vi "Link Parameters.vi"(7 "Virtual Memory Unit in":refnum<class "Virtual Memory Unit.lvclass">, 8 "error in (no error)":errorcluster, 11 "Remote Terminal in":refnum<class "Remote Terminal.lvclass">) -> (0 "error out":errorcluster, 3 "Remote Terminal out":refnum<class "Remote Terminal.lvclass">)   [LabVIEW 2020, in "BCI-1553 API.lvlib" / "Remote Terminal.lvclass"]
doc: "Should be the final configuration step. Actively links each parameter name to a base address that defines where the parameter may be located on the Holt IC. This is then stored in the appropriate Read/Write registries."
uses:
  Remote Terminal.lvclass
  Dependencies/Virtual Memory Unit/Virtual Memory Unit.lvclass
  Dependencies/Registry/Registry.lvclass/Registry.ctl
  Remote Terminal.lvclass/Remote Terminal.ctl
  <vilib>/Utility/error.llb/Clear Errors.vi
  Dependencies/Registry/Registry.lvclass
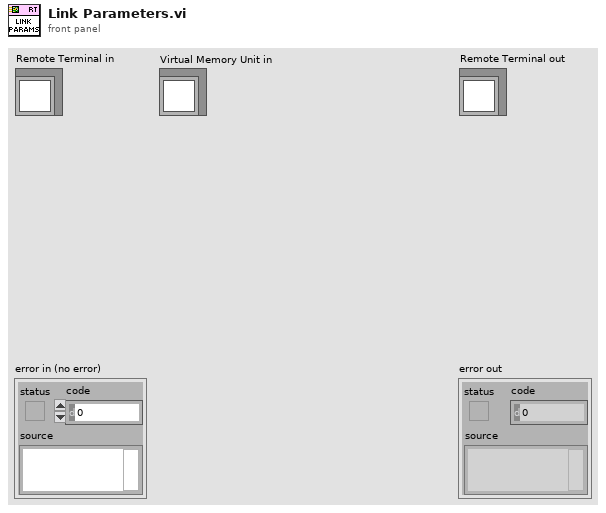
[diagram p1: front panel]
types:
  T1 = typedef "BCI-1553 API.lvlib/Remote Terminal.lvclass/RT CMD Config - Private.ctl" = cluster{"Command Type":T2, "SubAddress":T3, "Word Count\\Mode Code":T4, "Initial Data":u16[], "Data Fields":T5[]}
  T2 = typedef "BCI-1553 API.lvlib/Command Type.ctl" = enum16{"Transmit", "Receive"}
  T3 = typedef "BCI-1553 API.lvlib/Command SubAddress.ctl" = enum16{"Mode Code", "1", "2", "3", "4", "5", "6", "7", "8", "9", "10", "11", "12", "13", "14", "15", "16", "17", "18", "19", "20", "21", "22", "23", "24", "25", "26", "27", "28", "29", "30"}
  T4 = typedef "BCI-1553 API.lvlib/Command Word Count.ctl" = enum16{"1", "2", "3", "4", "5", "6", "7", "8", "9", "10", "11", "12", "13", "14", "15", "16", "17", "18", "19", "20", "21", "22", "23", "24", "25", "26", "27", "28", "29", "30", "31", "32"}
  T5 = typedef "BCI-1553 API.lvlib/Parameter Table Data.ctl" = cluster{"Parameter Name":string, "Base Word":u16, "Address":u16, "Value":u64, "Mask":u16[], "Scaling Info":T6}
  T6 = typedef "BCI-1553 API.lvlib/Scaling Information.ctl" = cluster{"Bit Offset":i32, "Bit Count":i32, "LSB Resolution":dbl, "2's Complement":bool, "Big Endian":bool, "Sign Bit":bool}
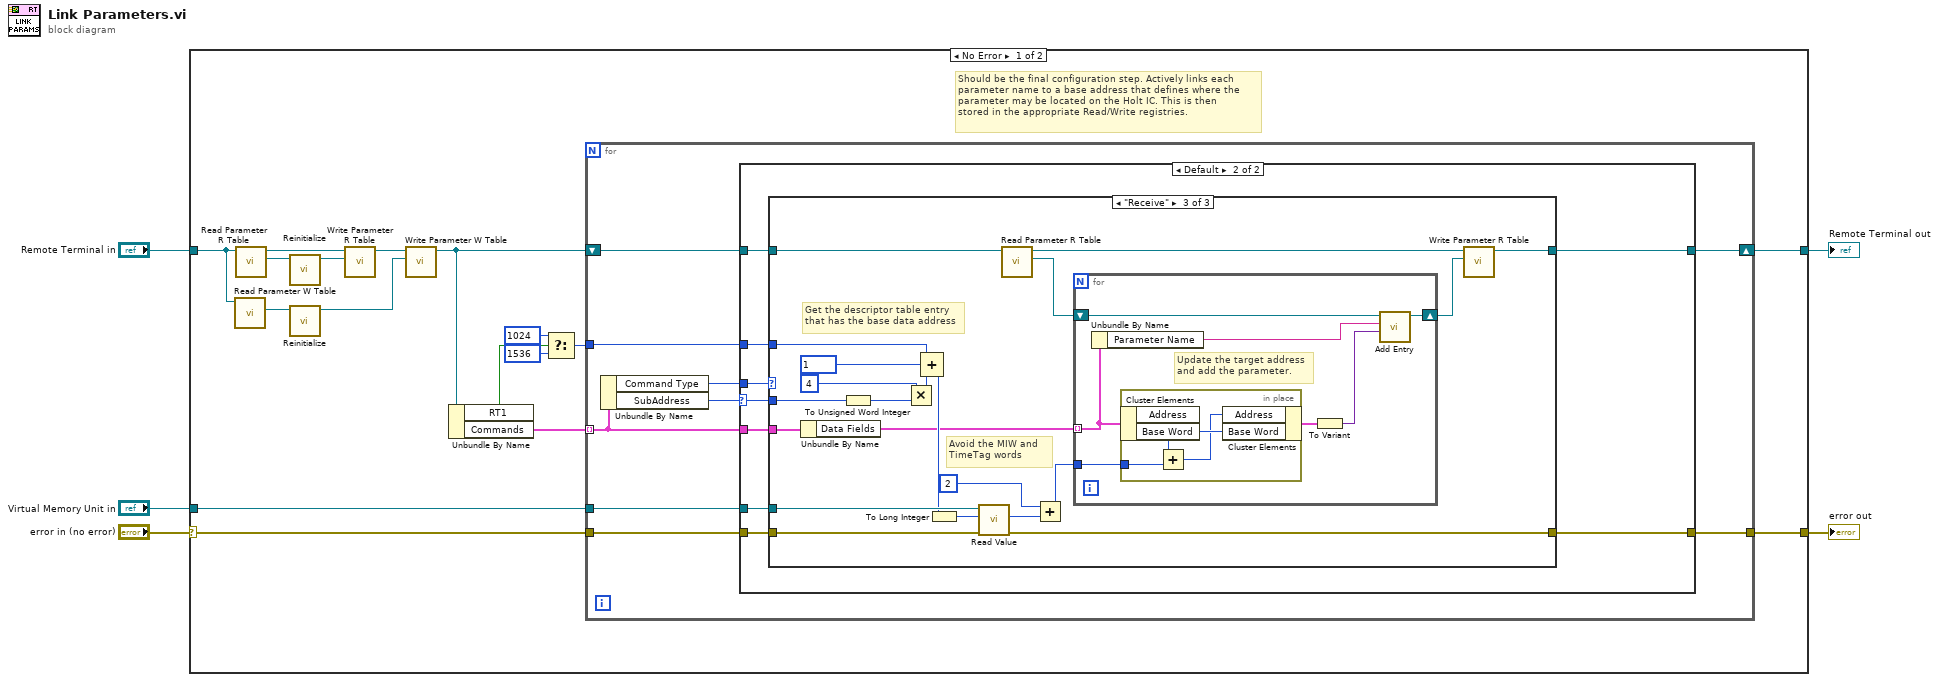
[diagram p0: block diagram]
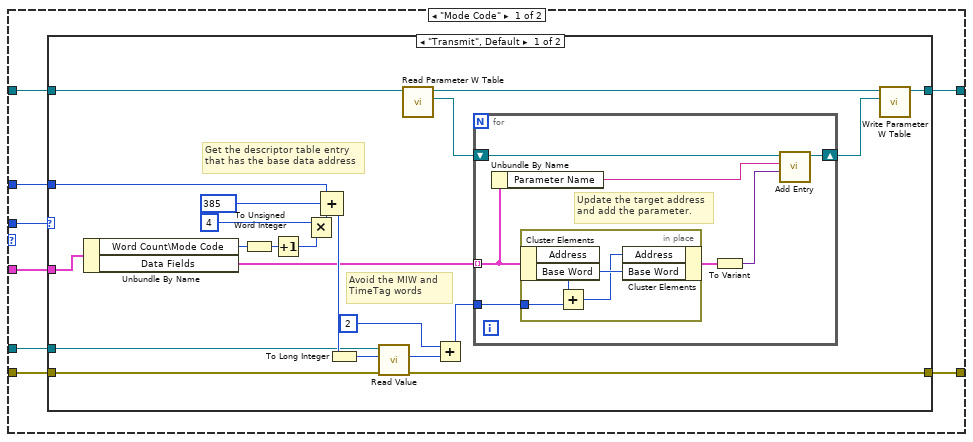
[diagram p2: hidden frame]
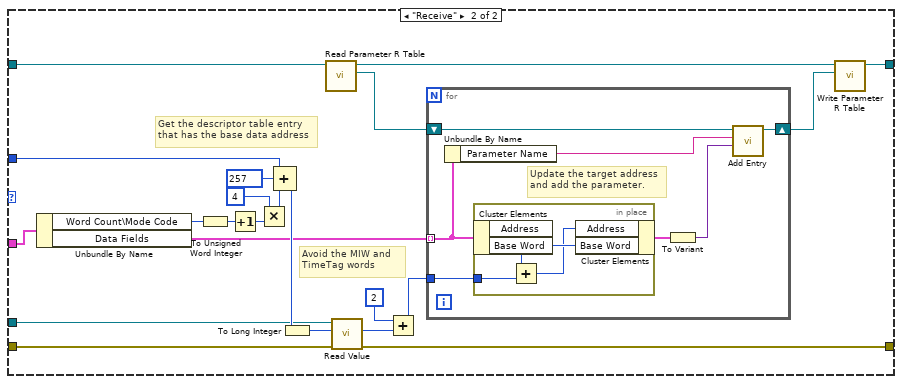
[diagram p3: hidden frame]
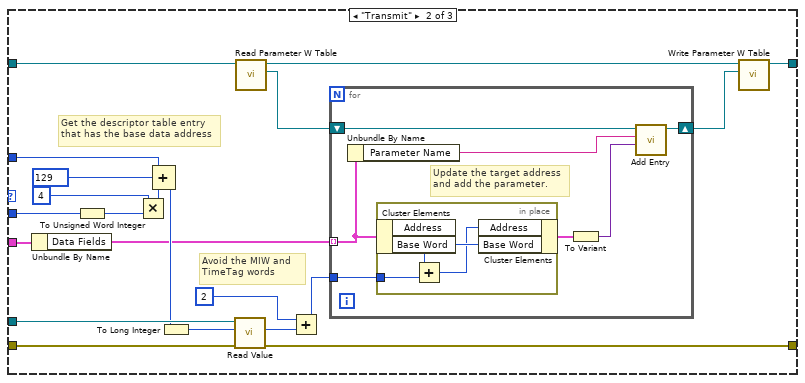
[diagram p5: hidden frame]
diagram:
  n1 = case shown="No Error" "error in (no error)" {
    selector: "error in (no error)" -> [w21 w178]
    tunnel: [w22 w178] -> w4
    tunnel: [w14 w177] -> w2
    tunnel: "Remote Terminal in" -> [w9 w177]
    tunnel: "Virtual Memory Unit in" -> [w20 _]
    frame No Error {
      # "Should be the final configuration step. Actively links each\nparameter name to a base address that defines where the\nparameter may be located on the Holt IC. This is then\nstored in the appropriate Read/Write registries."
      n2 = call-dynamic "Read Parameter W Table.vi"("1553 SubComponent in"=w9) -> ("Parameter W Table"=w10:refnum<class "Registry.lvclass">)  [unwired: 8 in, 2 out]
      n3 = call-dynamic "Read Parameter R Table.vi"("1553 SubComponent in"=w9) -> ("Parameter R Table"=w12:refnum<class "Registry.lvclass">, "1553 SubComponent out"=w13:refnum<class "Remote Terminal.lvclass">)  [unwired: 8 in, 1 out]
      n4 = call "Reinitialize.vi"("Registry in"=w12) -> ("Registry out"=w11:refnum<class "Registry.lvclass">)  [unwired: 9 in, 1 out]
      n5 = call "Reinitialize.vi"("Registry in"=w10) -> ("Registry out"=w6:refnum<class "Registry.lvclass">)  [unwired: 9 in, 1 out]
      n6 = call-dynamic "Write Parameter R Table.vi"("Parameter R Table"=w11, "1553 SubComponent in"=w13) -> ("1553 SubComponent out"=w8:refnum<class "Remote Terminal.lvclass">)  [unwired: 8 in, 1 out]
      n7 = call-dynamic "Write Parameter W Table.vi"("Parameter W Table"=w6, "1553 SubComponent in"=w8) -> ("1553 SubComponent out"=w7:refnum<class "Remote Terminal.lvclass">)  [unwired: 8 in, 1 out]
      n8 = Unbundle By Name(w7) -> ("RT1"=w15:bool, "Commands"=w19:T1[])
      n9 = Select(t=u16 1024 ("Address"), s=w15, f=u16 1536 ("Address")) -> (s? t:f=w16:u16)
      n10 = for {
        tunnel: w21 -> [w28]
        tunnel: [w29] -> w22
        tunnel: w19 -> [w30] mode=indexing
        tunnel: w16 -> [w26]
        tunnel: w20 -> [w27]
        shift-right: [w25] -> w14
        shift-left: w7 -> [w24]
        n11 = Unbundle By Name(w30) -> ("Command Type"=w31:T2, "SubAddress"=w23:T3)
        n12 = case shown="Default" w23 {
          selector: w23 -> [_ w104]
          tunnel: w31 -> [w35 w112]
          tunnel: w30 -> [w32 w111]
          tunnel: [w39 w110] -> w29
          tunnel: w28 -> [w38 w109]
          tunnel: w27 -> [w33 w108]
          tunnel: w26 -> [w34 w107]
          tunnel: [w37 w106] -> w25
          tunnel: w24 -> [w36 w105]
          frame "Mode Code" {
            n13 = case shown="\"Transmit\", Default" w35 {
              tunnel: [w42 w72] -> w39
              tunnel: w38 -> [w43 w73]
              tunnel: [w45 w75] -> w37
              tunnel: w36 -> [w46 w76]
              tunnel: w34 -> [w41 w77]
              tunnel: w33 -> [w44 w74]
              tunnel: w32 -> [w40 w78]
              frame "Transmit", Default {
                # "Get the descriptor table entry\nthat has the base data address"
                # "Avoid the MIW and\nTimeTag words"
                n14 = Unbundle By Name(w40) -> ("Word Count\\Mode Code"=w58:T4, "Data Fields"=w52:T5[])
                n15 = To Unsigned Word Integer(number=w58) -> (unsigned 16bit integer=w48:u16)
                n16 = Increment(x=w48) -> (x+1=w47:u16)
                n17 = Multiply(x=u16 4 ("y"), y=w47) -> (x*y=w59:u16)
                n18 = Compound Arithmetic op=ADD(w41, u16 385 ("Address"), w59) -> (w57:u16)
                n19 = To Long Integer(number=w57) -> (32bit integer=w56:i32)
                n20 = call "Read Value.vi"("error in (no error)"=w43, "Index"=w56, "Virtual Memory Unit in"=w44) -> ("error out"=w42:errorcluster, "Value"=w55:u16)  [unwired: 7 in]
                n21 = call-dynamic "Read Parameter W Table.vi"("1553 SubComponent in"=w46) -> ("Parameter W Table"=w50:refnum<class "Registry.lvclass">, "1553 SubComponent out"=w49:refnum<class "Remote Terminal.lvclass">)  [unwired: 8 in, 1 out]
                n22 = Add(x=u16 2 ("y"), y=w55) -> (x+y=w53:u16)
                n23 = for {
                  tunnel: w53 -> [w66]
                  tunnel: w52 -> [w65] mode=indexing
                  shift-right: [w67] -> w51
                  shift-left: w50 -> [w68]
                  # "Update the target address\nand add the parameter."
                  n24 = Unbundle By Name(w65) -> ("Parameter Name"=w64:string)
                  n25 = in-place {
                    in-place-border: w66 -> [w71]
                    n26 = in-place-cluster #1(w65) -> ("Base Word"=w70:u16)  [unwired: 1 out]
                    n27 = Add(x=w70, y=w71) -> (x+y=w69:u16)
                    n28 = in-place-cluster #1("Address"=w69, "Base Word"=w70) -> (w63:T5)
                  }
                  n29 = To Variant(anything=w63) -> (Variant=w62:variant)
                  n30 = call "Add Entry.vi"("Value"=w62, "Key"=w64, "Registry in"=w68) -> ("Registry out"=w67:refnum<class "Registry.lvclass">)  [unwired: 6 in, 2 out]
                }
                n31 = call-dynamic "Write Parameter W Table.vi"("Parameter W Table"=w51, "1553 SubComponent in"=w49) -> ("1553 SubComponent out"=w45:refnum<class "Remote Terminal.lvclass">)  [unwired: 8 in, 1 out]
              }
              frame "Receive" {
                # "Get the descriptor table entry\nthat has the base data address"
                # "Avoid the MIW and\nTimeTag words"
                n32 = Unbundle By Name(w78) -> ("Word Count\\Mode Code"=w90:T4, "Data Fields"=w84:T5[])
                n33 = To Unsigned Word Integer(number=w90) -> (unsigned 16bit integer=w80:u16)
                n34 = Increment(x=w80) -> (x+1=w79:u16)
                n35 = Multiply(x=u16 4 ("y"), y=w79) -> (x*y=w91:u16)
                n36 = Compound Arithmetic op=ADD(w77, u16 257 ("Address"), w91) -> (w89:u16)
                n37 = To Long Integer(number=w89) -> (32bit integer=w88:i32)
                n38 = call-dynamic "Read Parameter R Table.vi"("1553 SubComponent in"=w76) -> ("Parameter R Table"=w83:refnum<class "Registry.lvclass">, "1553 SubComponent out"=w82:refnum<class "Remote Terminal.lvclass">)  [unwired: 8 in, 1 out]
                n39 = call "Read Value.vi"("error in (no error)"=w73, "Index"=w88, "Virtual Memory Unit in"=w74) -> ("error out"=w72:errorcluster, "Value"=w87:u16)  [unwired: 7 in]
                n40 = Add(x=u16 2 ("y"), y=w87) -> (x+y=w85:u16)
                n41 = for {
                  tunnel: w85 -> [w98]
                  tunnel: w84 -> [w97] mode=indexing
                  shift-right: [w99] -> w81
                  shift-left: w83 -> [w100]
                  # "Update the target address\nand add the parameter."
                  n42 = Unbundle By Name(w97) -> ("Parameter Name"=w96:string)
                  n43 = in-place {
                    in-place-border: w98 -> [w103]
                    n44 = in-place-cluster #2(w97) -> ("Base Word"=w102:u16)  [unwired: 1 out]
                    n45 = Add(x=w102, y=w103) -> (x+y=w101:u16)
                    n46 = in-place-cluster #2("Address"=w101, "Base Word"=w102) -> (w95:T5)
                  }
                  n47 = To Variant(anything=w95) -> (Variant=w94:variant)
                  n48 = call "Add Entry.vi"("Value"=w94, "Key"=w96, "Registry in"=w100) -> ("Registry out"=w99:refnum<class "Registry.lvclass">)  [unwired: 6 in, 2 out]
                }
                n49 = call-dynamic "Write Parameter R Table.vi"("Parameter R Table"=w81, "1553 SubComponent in"=w82) -> ("1553 SubComponent out"=w75:refnum<class "Remote Terminal.lvclass">)  [unwired: 8 in, 1 out]
              }
            }
          }
          frame Default {
            n50 = case shown="\"Receive\"" w112 {
              tunnel: w111 -> [_ w135 w166]
              tunnel: [w114 w126 w157] -> w110
              tunnel: w109 -> [w114 w127 w158]
              tunnel: w108 -> [_ w130 w161]
              tunnel: w107 -> [_ w131 w162]
              tunnel: [w113 w119 w149] -> w106
              tunnel: w105 -> [w113 w122 w152]
              tunnel: w104 -> [_ w116 w147]
              frame Default {
              }
              frame "Transmit" {
                # "Get the descriptor table entry\nthat has the base data address"
                # "Avoid the MIW and\nTimeTag words"
                n51 = Unbundle By Name(w135) -> ("Data Fields"=w123:T5[])
                n52 = To Unsigned Word Integer(number=w116) -> (unsigned 16bit integer=w115:u16)
                n53 = Multiply(x=u16 4 ("y"), y=w115) -> (x*y=w132:u16)
                n54 = Compound Arithmetic op=ADD(w131, u16 129 ("Address"), w132) -> (w129:u16)
                n55 = To Long Integer(number=w129) -> (32bit integer=w128:i32)
                n56 = call "Read Value.vi"("error in (no error)"=w127, "Index"=w128, "Virtual Memory Unit in"=w130) -> ("error out"=w126:errorcluster, "Value"=w125:u16)  [unwired: 7 in]
                n57 = call-dynamic "Read Parameter W Table.vi"("1553 SubComponent in"=w122) -> ("Parameter W Table"=w121:refnum<class "Registry.lvclass">, "1553 SubComponent out"=w120:refnum<class "Remote Terminal.lvclass">)  [unwired: 8 in, 1 out]
                n58 = Add(x=u16 2 ("y"), y=w125) -> (x+y=w117:u16)
                n59 = for {
                  tunnel: w117 -> [w140]
                  tunnel: w123 -> [w139] mode=indexing
                  shift-right: [w141] -> w118
                  shift-left: w121 -> [w142]
                  # "Update the target address\nand add the parameter."
                  n60 = Unbundle By Name(w139) -> ("Parameter Name"=w138:string)
                  n61 = in-place {
                    in-place-border: w140 -> [w145]
                    n62 = in-place-cluster #3(w139) -> ("Base Word"=w144:u16)  [unwired: 1 out]
                    n63 = Add(x=w144, y=w145) -> (x+y=w143:u16)
                    n64 = in-place-cluster #3("Address"=w143, "Base Word"=w144) -> (w137:T5)
                  }
                  n65 = To Variant(anything=w137) -> (Variant=w136:variant)
                  n66 = call "Add Entry.vi"("Value"=w136, "Key"=w138, "Registry in"=w142) -> ("Registry out"=w141:refnum<class "Registry.lvclass">)  [unwired: 6 in, 2 out]
                }
                n67 = call-dynamic "Write Parameter W Table.vi"("Parameter W Table"=w118, "1553 SubComponent in"=w120) -> ("1553 SubComponent out"=w119:refnum<class "Remote Terminal.lvclass">)  [unwired: 8 in, 1 out]
              }
              frame "Receive" {
                # "Get the descriptor table entry\nthat has the base data address"
                # "Avoid the MIW and\nTimeTag words"
                n68 = Unbundle By Name(w166) -> ("Data Fields"=w153:T5[])
                n69 = To Unsigned Word Integer(number=w147) -> (unsigned 16bit integer=w146:u16)
                n70 = Multiply(x=u16 4 ("y"), y=w146) -> (x*y=w163:u16)
                n71 = Compound Arithmetic op=ADD(w162, u16 1 ("Address"), w163) -> (w160:u16)
                n72 = To Long Integer(number=w160) -> (32bit integer=w159:i32)
                n73 = call "Read Value.vi"("error in (no error)"=w158, "Index"=w159, "Virtual Memory Unit in"=w161) -> ("error out"=w157:errorcluster, "Value"=w156:u16)  [unwired: 7 in]
                n74 = call-dynamic "Read Parameter R Table.vi"("1553 SubComponent in"=w152) -> ("Parameter R Table"=w151:refnum<class "Registry.lvclass">, "1553 SubComponent out"=w150:refnum<class "Remote Terminal.lvclass">)  [unwired: 8 in, 1 out]
                n75 = Add(x=u16 2 ("y"), y=w156) -> (x+y=w154:u16)
                n76 = for {
                  tunnel: w154 -> [w171]
                  tunnel: w153 -> [w170] mode=indexing
                  shift-right: [w172] -> w148
                  shift-left: w151 -> [w173]
                  # "Update the target address\nand add the parameter."
                  n77 = Unbundle By Name(w170) -> ("Parameter Name"=w169:string)
                  n78 = in-place {
                    in-place-border: w171 -> [w176]
                    n79 = in-place-cluster #4(w170) -> ("Base Word"=w175:u16)  [unwired: 1 out]
                    n80 = Add(x=w175, y=w176) -> (x+y=w174:u16)
                    n81 = in-place-cluster #4("Address"=w174, "Base Word"=w175) -> (w168:T5)
                  }
                  n82 = To Variant(anything=w168) -> (Variant=w167:variant)
                  n83 = call "Add Entry.vi"("Value"=w167, "Key"=w169, "Registry in"=w173) -> ("Registry out"=w172:refnum<class "Registry.lvclass">)  [unwired: 6 in, 2 out]
                }
                n84 = call-dynamic "Write Parameter R Table.vi"("Parameter R Table"=w148, "1553 SubComponent in"=w150) -> ("1553 SubComponent out"=w149:refnum<class "Remote Terminal.lvclass">)  [unwired: 8 in, 1 out]
              }
            }
          }
        }
      }
    }
    frame Error {
    }
  }
  "error out" <- w4
  "Remote Terminal out" <- w2
